vi "Climber Teleop.vi"(11 "Buttons":bool[](array[boolean])) -> ()   [LabVIEW 2019]
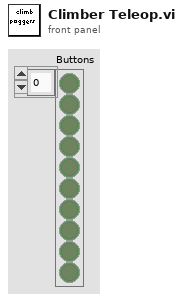
[diagram p1: front panel]
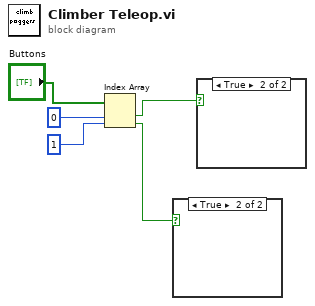
[diagram p0: block diagram]
diagram:
  n1 = Index Array(array="Buttons", index #1=0 ("index"), index #2=1 ("index")) -> (element #1=w2:bool, element #2=w1:bool)
  n2 = case shown="True" w1 {
    frame False {
    }
    frame True {
    }
  }
  n3 = case shown="True" w2 {
    frame False {
    }
    frame True {
    }
  }
